vi "VI Tree - array.vi"   [LabVIEW 2009]
uses:
  Reverse 2D Array/Reverse 2D Array (SGL).vi
  Slice 1D Array/Slice 1D Array (DBL).vi
  Sort Array/Sort 2D Array (DBL).vi
  Conditional Auto-Indexing Tunnel/Conditional Auto-Indexing Tunnel (DBL).vi
  Reorder Array/Reorder 2D Array (DBL).vi
  Empty Array/Empty 1D Array (DBL).vi
  Remove Duplicates from 1D Array/Remove Duplicates from 1D Array (DBL).vi
  Filter 1D Array/Filter 1D Array (DBL).vi
  Search Array/Search 1D Array (DBL).vi
  Sort Array/Sort 1D Array (DBL).vi
  Index Array Elements/Index 1D Array Elements (DBL).vi
  Delete Elements from Array/Delete Elements from 1D Array (DBL).vi
  Reorder Array/Reorder 2D Array2 (DBL).vi
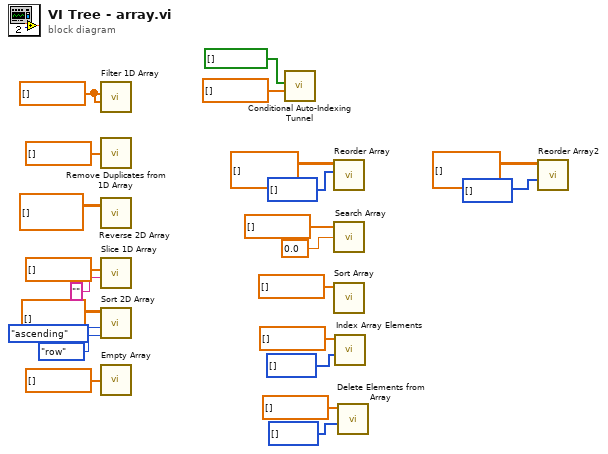
[diagram p0: block diagram]
diagram:
  w21 = dbl[] [] ("Array")
  n1 = call-poly "Filter 1D Array.vi"("items to filter"=w21, "array"=w21) -> ()  [unwired: 4 in, 2 out]
  n2 = call-poly "Remove Duplicates from 1D Array.vi"("Input Array"=dbl[] []) -> ()  [unwired: 2 out]
  n3 = call-poly "Reverse 2D Array.vi"("Array"=sgl[][] []) -> ()  [unwired: 2 in, 1 out]
  n4 = call-poly "Slice 1D Array.vi"("slice"="", "array"=dbl[] []) -> ()  [unwired: 5 in, 1 out]
  n5 = call-poly "Sort 2D Array.vi"("Sort By in"=enum16{"row", "column"}."row", "Order"=enum16{"ascending", "descending"}."ascending", "Array in"=dbl[][] []) -> ()  [unwired: 5 in, 4 out]
  n6 = call-poly "Empty Array.vi"("Array"=dbl[] []) -> ()  [unwired: 8 in, 1 out]
  n7 = call-poly "Conditional Auto-Indexing Tunnel.vi"("Array in"=dbl[] [], "Elements to keep"=bool[] []) -> ()  [unwired: 5 in, 1 out]
  n8 = call-poly "Reorder Array.vi"("Sorted Pointers in"=i32[] [], "Array in"=dbl[][] []) -> ()  [unwired: 7 in, 3 out]
  n9 = call-poly "Search Array.vi"("Array"=dbl[] [], "Element Data"=0.0) -> ()  [unwired: 7 in, 1 out]
  n10 = call-poly "Sort Array.vi"("Array in"=dbl[] []) -> ()  [unwired: 9 in, 2 out]
  n11 = call-poly "Index Array Elements.vi"("indices"=i32[] [], "array"=dbl[] []) -> ()  [unwired: 9 in, 1 out]
  n12 = call-poly "Delete Elements from Array.vi"("indices"=i32[] [], "array"=dbl[] []) -> ()  [unwired: 8 in, 2 out]
  n13 = call-poly "Reorder Array2.vi"("indices"=i32[] [] ("Sorted Pointers in"), "array"=dbl[][] [] ("Array in")) -> ()  [unwired: 9 in, 1 out]
